vi "Main Server.vi"() -> ()   [LabVIEW 2017]
uses:
  <vilib>/OPCUA/controls/Data Type.ctl
  <vilib>/OPCUA/controls/Supported Security Policies.ctl
  <vilib>/OPCUA/server/Read Bool Array.vi
  <vilib>/OPCUA/NI OPC UA Server.lvlib
  <vilib>/OPCUA/NI OPC UA Utility.lvlib
panel:
  out "MATLAB Booleans Node":string
  out "BoP Output Node":string
  out "BoP Input Node":string
  out "Result Boolean Control Node":string
  out "Result Numeric Control Node":string
  out "Result Data Node":string
  out "Spoof Boolean Control Node":string
  out "Spoof Numeric Control Node":string
  out "Spoof Data Node":string
  out "Chat Node":string
  out "Boolean Control Action Node":string
  out "Numeric Control Action Node":string
  out "certificate path 2":path
  out "certificate path":path
  out "error out":errorcluster
  out "CIET Data Node":string
  out "server endpoint URL":string
  in  "Stop":bool
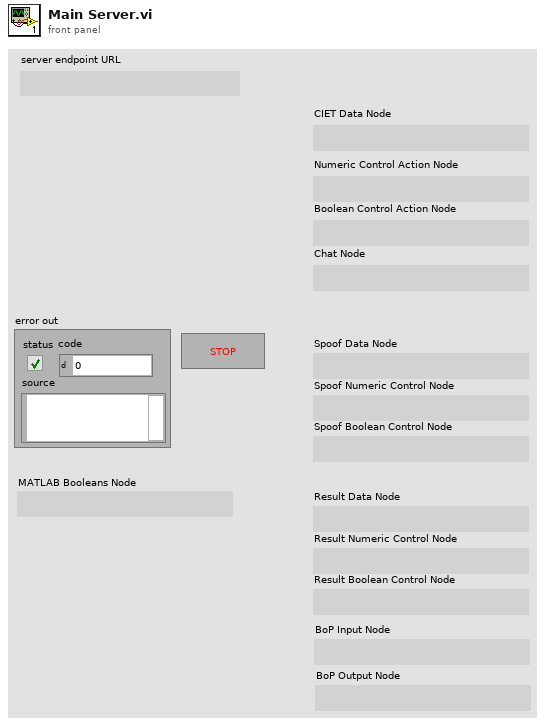
[diagram p1: front panel]
types:
  T1 = typedef "Data Type.ctl" = u16
  T2 = cluster{"name":string, "data type":T1, "access level":u16, "description":string}
  T3 = cluster{"name":string, "data type":T1, "access level 2":u16, "description":string}
  T4 = typedef "Supported Security Policies.ctl" = cluster{"None":bool, "Sign with Basic128Rsa15":bool, "Sign and Encrypt with Basic128Rsa15":bool, "Sign with Basic256":bool, "Sign and Encrypt with Basic256":bool}
  T5 = typedef "OPC UA Server Refnum.ctl" = refnum<k21>
  T6 = typedef "NodeId.ctl" = string
  T7 = cluster{"value[0]":bool, "value[1]":bool, "value[2]":bool, "value[3]":bool, "value[4]":bool, "value[5]":bool, "value[6]":bool, "value[7]":bool, "value[8]":bool}
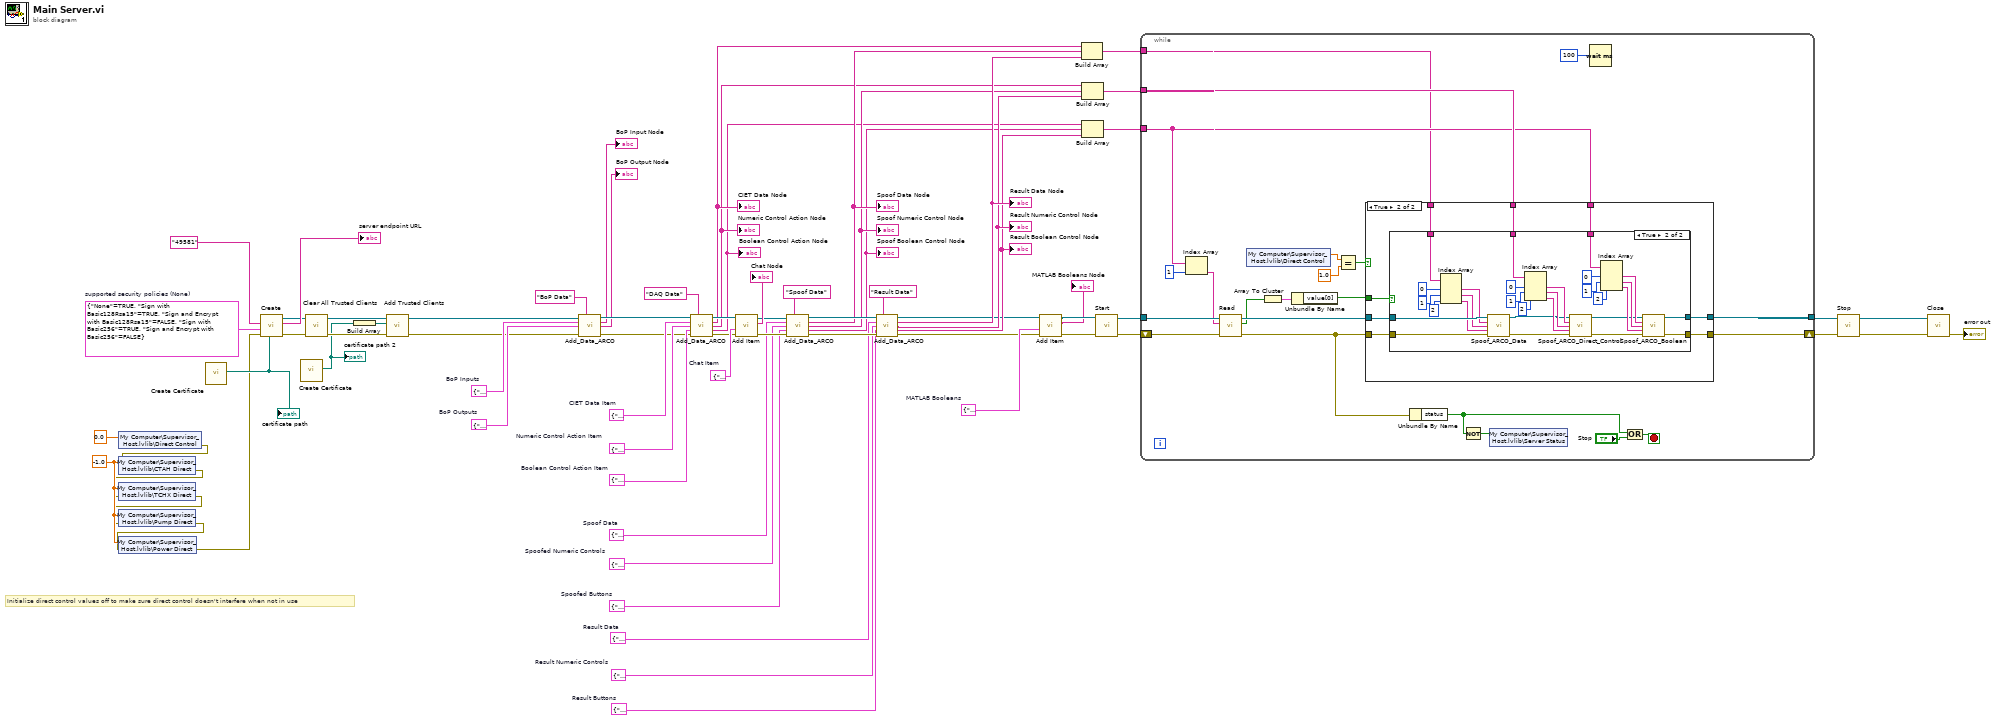
[diagram p0: block diagram]
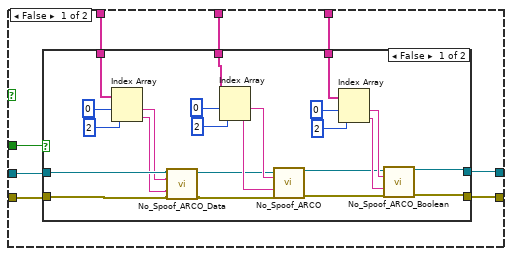
[diagram p2: hidden frame]
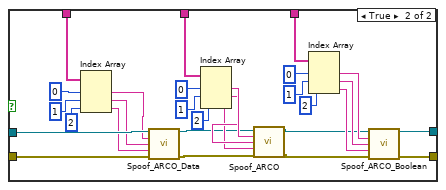
[diagram p3: hidden frame]
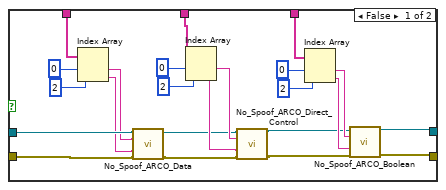
[diagram p4: hidden frame]
diagram:
  w11 = T2 {"name"="MATLAB Booleans", "data type"=101, "access level"=3, "description"="Controls to start and stop MATLAB routines"}  # MATLAB Booleans
  w12 = sgl -1.0 ("CTAH Direct")
  w20 = T2 {"name"="BoP Outputs", "data type"=111, "access level"=3, "description"="BoP Output Values"}  # BoP Outputs
  w21 = T2 {"name"="BoP Inputs", "data type"=111, "access level"=3, "description"="BoP Input Values"}  # BoP Inputs
  w38 = T2 {"name"="Spoofed Numeric Controls", "data type"=111, "access level"=3, "description"="Spoofed Setpoints"}  # Spoofed Numeric Controls
  w39 = T2 {"name"="Spoofed CIET Data", "data type"=111, "access level"=3, "description"="Spoofed CIET TC and FM"}  # Spoof Data
  w42 = T2 {"name"="Result Boolean Controls", "data type"=101, "access level"=3, "description"="Result Buttons"}  # Result Buttons
  w43 = T2 {"name"="Result Numeric Controls", "data type"=111, "access level"=3, "description"="Result Setpoints"}  # Result Numeric Controls
  w44 = T3 {"name"="Result CIET Data", "data type"=111, "access level 2"=3, "description"="Result CIET TC and FM"}  # Result Data
  w37 = T2 {"name"="Spoofed Boolean Controls", "data type"=101, "access level"=3, "description"="Spoofed Buttons"}  # Spoofed Buttons
  w56 = T2 {"name"="Chat", "data type"=12, "access level"=3, "description"="Chat"}  # Chat Item
  w52 = T2 {"name"="Boolean Control Actions", "data type"=101, "access level"=3, "description"="Buttons"}  # Boolean Control Action Item
  w53 = T2 {"name"="Numeric Control Actions", "data type"=111, "access level"=3, "description"="Setpoints"}  # Numeric Control Action Item
  w65 = T4 {"None"=TRUE, "Sign with Basic128Rsa15"=TRUE, "Sign and Encrypt with Basic128Rsa15"=FALSE, "Sign with Basic256"=TRUE, "Sign and Encrypt with Basic256"=FALSE}  # supported security policies (None)
  w54 = T2 {"name"="CIET Data", "data type"=111, "access level"=3, "description"="CIET TC and FM"}  # CIET Data Item
  # "Initialize direct control values off to make sure direct control doesn't interfere when not in use"
  n1 = shared-variable "My Computer\\Supervisor_Host.lvlib\\Direct Control"(sgl 0.0 ("Direct Control")) -> (error out=w5:errorcluster)  [unwired: 1 in]
  n2 = shared-variable "My Computer\\Supervisor_Host.lvlib\\CTAH Direct"(w12, error in=w5) -> (error out=w4:errorcluster)
  n3 = shared-variable "My Computer\\Supervisor_Host.lvlib\\TCHX Direct"(w12, error in=w4) -> (error out=w3:errorcluster)
  n4 = shared-variable "My Computer\\Supervisor_Host.lvlib\\Pump Direct"(w12, error in=w3) -> (error out=w2:errorcluster)
  n5 = shared-variable "My Computer\\Supervisor_Host.lvlib\\Power Direct"(w12, error in=w2) -> (error out=w1:errorcluster)
  n6 = call <vilib>:"Create Certificate.vi"() -> ("certificate path"=w60:path)  [unwired: 8 in, 3 out]
  "certificate path" <- w60
  n7 = call <vilib>:"Create.vi"("server certificate file"=w60, "error in (no error)"=w1, "supported security policies (None)"=w65, "TCP port (49580)"="49581") -> ("error out"=w61:errorcluster, "server endpoint URL"=→"server endpoint URL":string, "OPC UA server refnum out"=w62:T5)  [unwired: 5 in]
  n8 = call <vilib>:"Create Certificate.vi"() -> ("certificate path"=w59:path)  [unwired: 8 in, 3 out]
  "certificate path 2" <- w59
  n9 = call <vilib>:"Clear All Trusted Clients.vi"("error in (no error)"=w61, "OPC UA server refnum in"=w62) -> ("error out"=w63:errorcluster, "OPC UA server refnum out"=w64:T5)  [unwired: 8 in]
  n10 = Build Array(w59) -> (w58:path[])
  n11 = call <vilib>:"Add Trusted Clients.vi"("error in (no error)"=w63, "trusted client certificates"=w58, "OPC UA server refnum in"=w64) -> ("error out"=w18:errorcluster, "OPC UA server refnum out"=w19:T5)  [unwired: 7 in]
  n12 = call "Add_Data_ARCO.vi"("Refnum in"=w19, "folder name"="BoP Data", "item 1"=w21, "item 2"=w20, "error in (no error)"=w18) -> ("Refnum out"=w16:T5, "item node ID 1"=→"BoP Input Node":string, "item node ID 2"=→"BoP Output Node":string, "error out"=w17:errorcluster)  [unwired: 6 in, 1 out]
  n13 = call "Add_Data_ARCO.vi"("Refnum in"=w16, "folder name"="DAQ Data", "item 1"=w54, "item 2"=w53, "item 3"=w52, "error in (no error)"=w17) -> ("Refnum out"=w51:T5, "item node ID 1"=w33:string, "item node ID 2"=w30:string, "item node ID 3"=w27:string, "error out"=w50:errorcluster)  [unwired: 5 in]
  "CIET Data Node" <- w33
  "Numeric Control Action Node" <- w30
  "Boolean Control Action Node" <- w27
  n14 = call <vilib>:"Add Item.vi"("error in (no error)"=w50, "item"=w56, "OPC UA server refnum in"=w51) -> ("error out"=w47:errorcluster, "item node ID"=→"Chat Node":T6, "OPC UA server refnum out"=w48:T5)  [unwired: 4 in, 1 out]
  n15 = call "Add_Data_ARCO.vi"("Refnum in"=w48, "folder name"="Spoof Data", "item 1"=w39, "item 2"=w38, "item 3"=w37, "error in (no error)"=w47) -> ("Refnum out"=w45:T5, "item node ID 1"=w32:string, "item node ID 2"=w29:string, "item node ID 3"=w26:string, "error out"=w46:errorcluster)  [unwired: 5 in]
  "Spoof Data Node" <- w32
  "Spoof Numeric Control Node" <- w29
  "Spoof Boolean Control Node" <- w26
  n16 = call "Add_Data_ARCO.vi"("Refnum in"=w45, "folder name"="Result Data", "item 1"=w44, "item 2"=w43, "item 3"=w42, "error in (no error)"=w46) -> ("Refnum out"=w6:T5, "item node ID 1"=w31:string, "item node ID 2"=w28:string, "item node ID 3"=w25:string, "error out"=w10:errorcluster)  [unwired: 5 in]
  "Result Data Node" <- w31
  "Result Numeric Control Node" <- w28
  "Result Boolean Control Node" <- w25
  n17 = call <vilib>:"Add Item.vi"("error in (no error)"=w10, "item"=w11, "OPC UA server refnum in"=w6) -> ("error out"=w9:errorcluster, "item node ID"=→"MATLAB Booleans Node":T6, "OPC UA server refnum out"=w8:T5)  [unwired: 4 in, 1 out]
  n18 = Build Array(w33, w32, w31) -> (w36:string[])
  n19 = Build Array(w30, w29, w28) -> (w35:string[])
  n20 = Build Array(w27, w26, w25) -> (w34:string[])
  n21 = call <vilib>:"Start.vi"("error in (no error)"=w9, "OPC UA server refnum in"=w8) -> ("error out"=w24:errorcluster, "OPC UA server refnum out"=w70:T5)  [unwired: 7 in, 1 out]
  n22 = while {
    tunnel: [w92] -> w69
    tunnel: w70 -> [w85]
    tunnel: w36 -> [w75]
    tunnel: w35 -> [w81]
    tunnel: w34 -> [w76]
    shift-right: [w90] -> w23
    shift-left: w24 -> [w86]
    stop <- w89 stop-if-true
    n23 = Index Array(array=w76, index=1) -> (element=w80:string)
    n24 = call-poly <vilib>:"Read.vi"("error in (no error)"=w86, "node ID"=w80, "OPC UA server refnum in"=w85) -> ("error out"=w83:errorcluster, "value"=w79:bool[], "OPC UA server refnum out"=w84:T5)  [unwired: 4 in, 2 out]
    n25 = shared-variable "My Computer\\Supervisor_Host.lvlib\\Direct Control"() -> (w74:sgl)  [unwired: 1 in, 1 out]
    n26 = Array To Cluster(array=w79) -> (cluster=w78:T7)
    n27 = Unbundle By Name(w78) -> ("value[0]"=w77:bool)
    n28 = Equal?(x=w74, y=sgl 1.0) -> (x = y?=w72:bool)
    n29 = case shown="True" w72 {
      tunnel: [w96 w161] -> w92
      tunnel: [w95 w160] -> w90
      tunnel: w84 -> [w98 w159]
      tunnel: w83 -> [w97 w158]
      tunnel: w81 -> [w100 w157]
      tunnel: w77 -> [w94 w156]
      tunnel: w76 -> [w99 w155]
      tunnel: w75 -> [w101 w154]
      frame False {
        n30 = case shown="False" w94 {
          tunnel: [w110 w153] -> w96
          tunnel: w98 -> [w104 w128]
          tunnel: w100 -> [w113 w140]
          tunnel: w99 -> [w118 w139]
          tunnel: [w109 w138] -> w95
          tunnel: w97 -> [w105 w129]
          tunnel: w101 -> [w108 w132]
          frame False {
            n31 = Index Array(array=w108, index #1=0, index #2=2 ("index")) -> (element #1=w103:string, element #2=w102:string)
            n32 = call "No_Spoof_ARCO_Data.vi"("OPC UA server refnum in"=w104, "DAQ Node"=w103, "Result Node"=w102, "error in (no error)"=w105) -> ("OPC UA server refnum out"=w107:T5, "error out"=w106:errorcluster)  [unwired: 10 in]
            n33 = Index Array(array=w113, index #1=0, index #2=2 ("index")) -> (element #1=w115:string, element #2=w114:string)
            n34 = call "No_Spoof_ARCO.vi"("OPC UA server refnum in"=w107, "DAQ Node"=w115, "Result Node"=w114, "error in (no error)"=w106) -> ("OPC UA server refnum out"=w112:T5, "error out"=w111:errorcluster)  [unwired: 10 in]
            n35 = Index Array(array=w118, index #1=0, index #2=2 ("index")) -> (element #1=w120:string, element #2=w119:string)
            n36 = call "No_Spoof_ARCO_Boolean.vi"("OPC UA server refnum in"=w112, "DAQ Node"=w120, "Result Node"=w119, "error in (no error)"=w111) -> ("OPC UA server refnum out"=w110:T5, "error out"=w109:errorcluster)  [unwired: 10 in]
          }
          frame True {
            n37 = Index Array(array=w132, index #1=0, index #2=1, index #3=2) -> (element #1=w125:string, element #2=w126:string, element #3=w127:string)
            n38 = call "Spoof_ARCO_Data.vi"("OPC UA server refnum in"=w128, "DAQ Node"=w125, "Spoof Node"=w126, "Result Node"=w127, "error in (no error)"=w129) -> ("OPC UA server refnum out"=w131:T5, "error out"=w130:errorcluster)  [unwired: 9 in]
            n39 = Index Array(array=w140, index #1=0, index #2=1, index #3=2) -> (element #1=w137:string, element #2=w136:string, element #3=w135:string)
            n40 = call "Spoof_ARCO.vi"("OPC UA server refnum in"=w131, "DAQ Node"=w137, "Spoof Node"=w136, "Result Node"=w135, "error in (no error)"=w130) -> ("OPC UA server refnum out"=w134:T5, "error out"=w133:errorcluster)  [unwired: 9 in]
            n41 = Index Array(array=w139, index #1=0, index #2=1, index #3=2) -> (element #1=w141:string, element #2=w142:string, element #3=w143:string)
            n42 = call "Spoof_ARCO_Boolean.vi"("OPC UA server refnum in"=w134, "DAQ Node"=w141, "Spoof Node"=w142, "Result Node"=w143, "error in (no error)"=w133) -> ("OPC UA server refnum out"=w153:T5, "error out"=w138:errorcluster)  [unwired: 9 in]
          }
        }
      }
      frame True {
        n43 = case shown="True" w156 {
          tunnel: [w174 w213] -> w161
          tunnel: w159 -> [w170 w195]
          tunnel: w157 -> [w175 w200]
          tunnel: w155 -> [w178 w199]
          tunnel: [w173 w198] -> w160
          tunnel: w158 -> [w171 w196]
          tunnel: w154 -> [w172 w197]
          frame False {
            n44 = Index Array(array=w172, index #1=0, index #2=2 ("index")) -> (element #1=w169:string, element #2=w168:string)
            n45 = call "No_Spoof_ARCO_Data.vi"("OPC UA server refnum in"=w170, "DAQ Node"=w169, "Result Node"=w168, "error in (no error)"=w171) -> ("OPC UA server refnum out"=w162:T5, "error out"=w165:errorcluster)  [unwired: 10 in]
            n46 = Index Array(array=w175, index #1=0, index #2=2 ("index")) -> (element #1=w163:string, element #2=w164:string)
            n47 = call "No_Spoof_ARCO_Direct_Control.vi"("OPC UA server refnum in"=w162, "DAQ Node"=w163, "Result Node"=w164, "error in (no error)"=w165) -> ("OPC UA server refnum out"=w167:T5, "error out"=w166:errorcluster)  [unwired: 10 in]
            n48 = Index Array(array=w178, index #1=0, index #2=2 ("index")) -> (element #1=w180:string, element #2=w179:string)
            n49 = call "No_Spoof_ARCO_Boolean.vi"("OPC UA server refnum in"=w167, "DAQ Node"=w180, "Result Node"=w179, "error in (no error)"=w166) -> ("OPC UA server refnum out"=w174:T5, "error out"=w173:errorcluster)  [unwired: 10 in]
          }
          frame True {
            n50 = Index Array(array=w197, index #1=0, index #2=1, index #3=2) -> (element #1=w192:string, element #2=w193:string, element #3=w194:string)
            n51 = call "Spoof_ARCO_Data.vi"("OPC UA server refnum in"=w195, "DAQ Node"=w192, "Spoof Node"=w193, "Result Node"=w194, "error in (no error)"=w196) -> ("OPC UA server refnum out"=w185:T5, "error out"=w189:errorcluster)  [unwired: 9 in]
            n52 = Index Array(array=w200, index #1=0, index #2=1, index #3=2) -> (element #1=w186:string, element #2=w187:string, element #3=w188:string)
            n53 = call "Spoof_ARCO_Direct_Control.vi"("OPC UA server refnum in"=w185, "DAQ Node"=w186, "Spoof Node"=w187, "Result Node"=w188, "error in (no error)"=w189) -> ("OPC UA server refnum out"=w191:T5, "error out"=w190:errorcluster)  [unwired: 9 in]
            n54 = Index Array(array=w199, index #1=0, index #2=1, index #3=2) -> (element #1=w201:string, element #2=w202:string, element #3=w203:string)
            n55 = call "Spoof_ARCO_Boolean.vi"("OPC UA server refnum in"=w191, "DAQ Node"=w201, "Spoof Node"=w202, "Result Node"=w203, "error in (no error)"=w190) -> ("OPC UA server refnum out"=w213:T5, "error out"=w198:errorcluster)  [unwired: 9 in]
          }
        }
      }
    }
    n56 = Unbundle By Name(w83) -> ("status"=w87:bool)
    n57 = Not(x=w87) -> (.not. x?=w91:bool)
    n58 = shared-variable "My Computer\\Supervisor_Host.lvlib\\Server Status"(w91) -> ()  [unwired: 1 in, 1 out]
    n59 = Wait (ms)(milliseconds to wait=u32 100) -> ()  [unwired: 1 out]
    n60 = Or(x=w87, y="Stop") -> (x .or. y?=w89:bool)
  }
  n61 = call <vilib>:"Stop.vi"("error in (no error)"=w23, "OPC UA server refnum in"=w69) -> ("error out"=w67:errorcluster, "OPC UA server refnum out"=w68:T5)  [unwired: 8 in]
  n62 = call <vilib>:"Close.vi"("error in (no error)"=w67, "OPC UA server refnum in"=w68) -> ("error out"=→"error out":errorcluster)  [unwired: 9 in]
